vi "TestPosCon.vi"() -> ()   [LabVIEW 2020]
doc: "Test program for Edge On"
panel:
  out "Waveform Chart":cluster{"Error":dbl, "OutputValue":dbl}(graph)
  out "UnfilteredOnTarget":bool
  in  "ConsecutiveTargets":dbl
  in  "Threshold":dbl
  in  "MaxDemand":dbl
  in  "MinDemand":dbl
  in  "Error":dbl
  in  "Deadband":dbl
  out "Output":dbl
  out "count":i32
  out "OnTarget?":bool
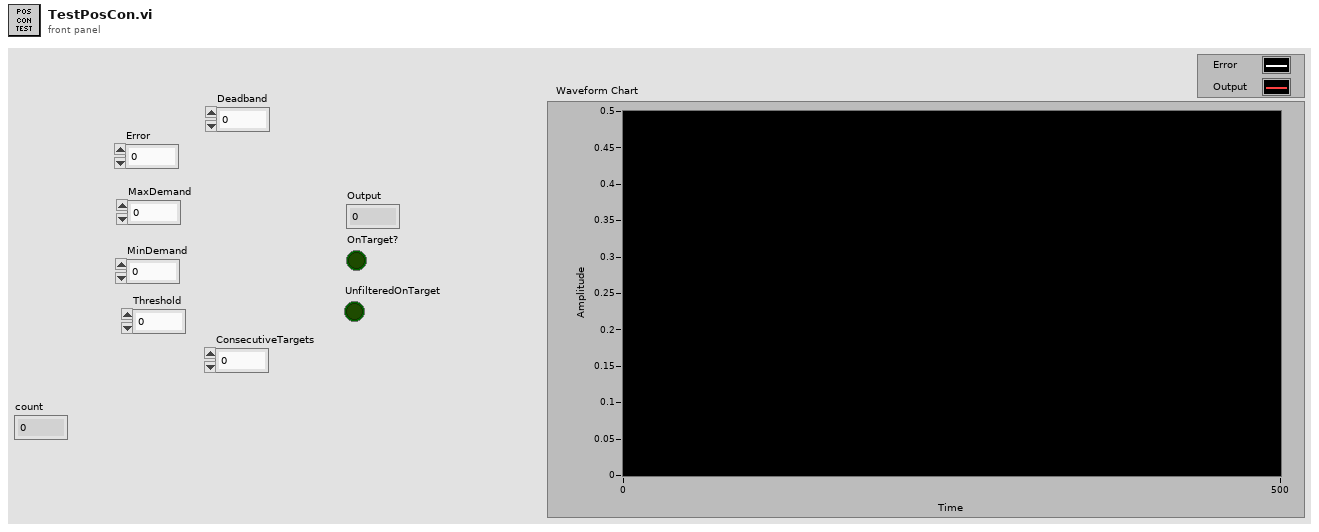
[diagram p1: front panel]
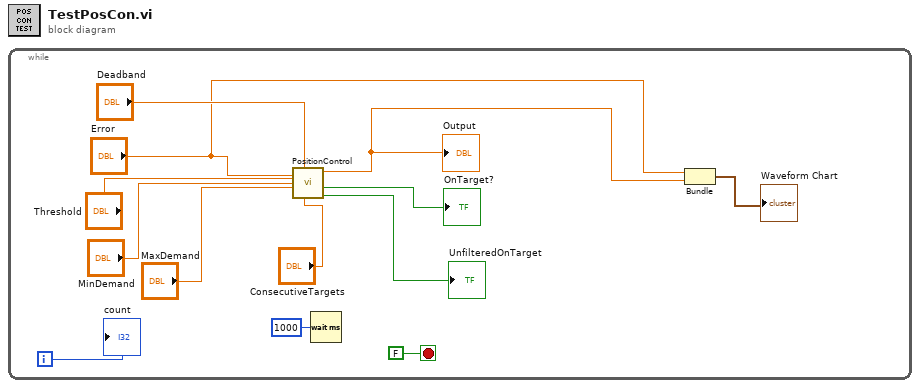
[diagram p0: block diagram]
diagram:
  n1 = while {
    i -> [w11]
    stop <- FALSE stop-if-true
    n2 = call "PositionControl.vi"("ConsecutiveTargets"="ConsecutiveTargets", "ErrorDeadband"="Deadband", "MaxOutput"="Threshold", "MinOutput"="MaxDemand", "ErrorThreshold"="MinDemand", "Error"="Error") -> ("UnfilteredOnTarget"=→"UnfilteredOnTarget":bool, "OnTarget"=→"OnTarget?":bool, "OutputValue"=w2:dbl)  [unwired: 3 in]
    "Output" <- w2
    n3 = Wait (ms)(milliseconds to wait=u32 1000) -> ()  [unwired: 1 out]
    n4 = Bundle("Error"="Error", "OutputValue"=w2) -> (→"Waveform Chart":cluster{"Error":dbl, "OutputValue":dbl})  [unwired: 1 in]
    "count" <- w11
  }
